vi "Polygon Centroid.vi"(10 "Y":dbl[](array[numeric]), 11 "X":dbl[](array[numeric])) -> (0 "error":i32, 2 "Centroid Y":dbl, 3 "Centroid X":dbl)   [LabVIEW 2017, in "NI_AAL_Geometry.lvlib"]
doc: "Computes the centroid of a polygon."
uses:
  <vilib>/Analysis/NI_AAL_Geometry.lvlib
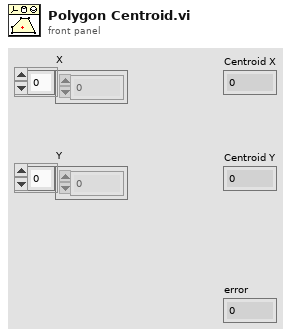
[diagram p1: front panel]
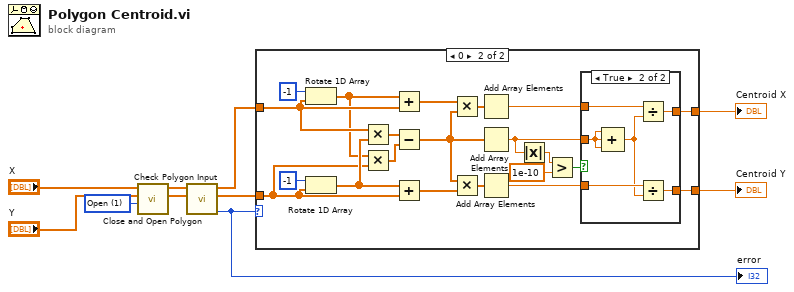
[diagram p0: block diagram]
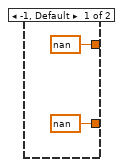
[diagram p2: hidden frame]
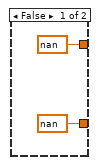
[diagram p3: hidden frame]
diagram:
  w8 = u16 1 items=["Closed", "Open"] ("type")
  n1 = call <vilib>:"Close and Open Polygon.vi"("type"=w8, "Y In"="Y", "X In"="X") -> ("Y Out"=w6:dbl[], "X Out"=w7:dbl[])  [unwired: 7 in]
  n2 = call <vilib>:"Check Polygon Input.vi"("Y In"=w6, "X In"=w7) -> ("error"=w1:i32, "Y Out"=w10:dbl[], "X Out"=w9:dbl[])  [unwired: 7 in]
  "error" <- w1
  n3 = case shown="0" w1 {
    tunnel: w9 -> [_ w31]
    tunnel: w10 -> [_ w26]
    tunnel: [nan w18] -> w3
    tunnel: [nan w17] -> w2
    frame -1, Default {
    }
    frame 0 {
      n4 = Rotate 1D Array(1:w31, 2:-1 ("n")) -> (0:w29:dbl[])
      n5 = Rotate 1D Array(1:w26, 2:-1 ("n")) -> (0:w30:dbl[])
      n6 = Multiply(x=w31, y=w30) -> (x*y=w28:dbl[])
      n7 = Multiply(x=w29, y=w26) -> (x*y=w27:dbl[])
      n8 = Add(x=w29, y=w31) -> (x+y=w25:dbl[])
      n9 = Subtract(x=w28, y=w27) -> (x-y=w21:dbl[])
      n10 = Add(x=w30, y=w26) -> (x+y=w24:dbl[])
      n11 = Multiply(x=w25, y=w21) -> (x*y=w23:dbl[])
      n12 = Multiply(x=w21, y=w24) -> (x*y=w22:dbl[])
      n13 = Add Array Elements(numeric array=w23) -> (sum=w20:dbl)
      n14 = Add Array Elements(numeric array=w21) -> (sum=w16:dbl)
      n15 = Add Array Elements(numeric array=w22) -> (sum=w19:dbl)
      n16 = Absolute Value(x=w16) -> (abs(x)=w15:dbl)
      n17 = Greater?(x=w15, y=1e-10) -> (0:w14:bool)
      n18 = case shown="True" w14 {
        tunnel: w20 -> [_ w41]
        tunnel: w19 -> [_ w40]
        tunnel: w16 -> [_ w39]
        tunnel: [nan w37] -> w18
        tunnel: [nan w36] -> w17
        frame False {
        }
        frame True {
          n19 = Compound Arithmetic op=ADD(w39, w39, w39) -> (w38:dbl)
          n20 = Divide(x=w41, y=w38) -> (x/y=w37:dbl)
          n21 = Divide(x=w40, y=w38) -> (x/y=w36:dbl)
        }
      }
    }
  }
  "Centroid X" <- w3
  "Centroid Y" <- w2
